vi "Install XNET and Scan If Needed.vi"(4 "XNET available":bool, 6 "xnet software to install":T1[](array[typedef]) {"component type" items=["standard", "hidden", "system", "unknown", "startup", "image"]}, 8 "error in (no error)":errorcluster, 9 "scan software to install":T1[](array[typedef]) {"component type" items=["standard", "hidden", "system", "unknown", "startup", "image"]}, 10 "software components on target":T1[](array[typedef]) {"component type" items=["standard", "hidden", "system", "unknown", "startup", "image"]}, 11 "Refnum in":refnum<k21>) -> (0 "error out":errorcluster, 3 "Refnum out":refnum<k21>)   [LabVIEW 2013]
uses:
  <vilib>/nisyscfg/Software 1.2.ctl
  <vilib>/nisyscfg/Component Type.ctl
  <vilib>/nisyscfg/Install or Uninstall Components.vi
  <vilib>/nisyscfg/Get Installed Components.vi
  <vilib>/nisyscfg/nisyscfg.lvlib
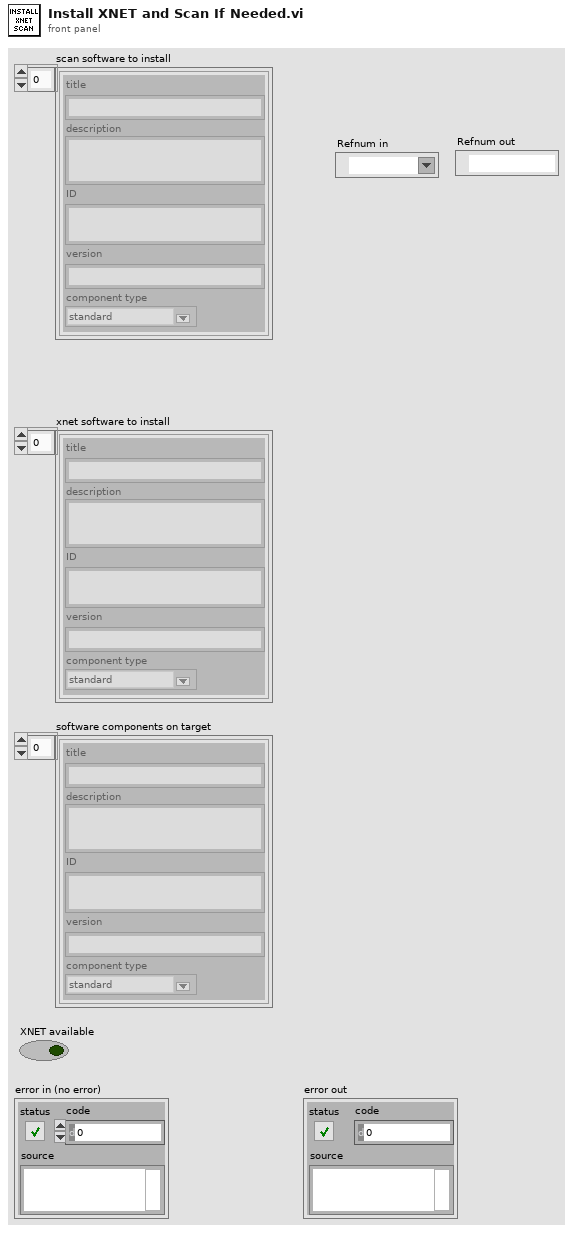
[diagram p1: front panel]
types:
  T1 = typedef "nisyscfg.lvlib/Software 1.2.ctl" = cluster{"title":string, "description":string, "ID":string, "version":string, "component type":T2}
  T2 = typedef "nisyscfg.lvlib/Component Type.ctl" = u32
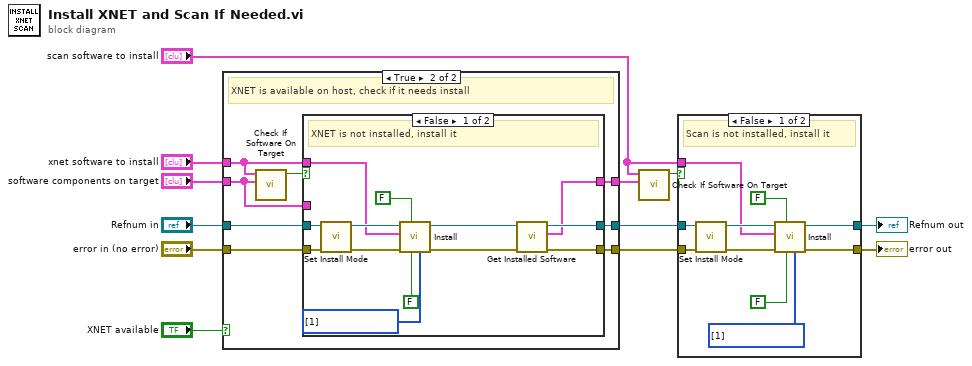
[diagram p0: block diagram]
diagram:
  n1 = case shown="True" "XNET available" {
    tunnel: "software components on target" -> [w13 w16]
    tunnel: "xnet software to install" -> [_ w20]
    tunnel: "error in (no error)" -> [w14 w22]
    tunnel: "Refnum in" -> [w15 w21]
    tunnel: [w14 w19] -> w9
    tunnel: [w15 w18] -> w6
    tunnel: [w13 w17] -> w1
    frame False {
      # "XNET not avilable on host, skip it"
    }
    frame True {
      # "XNET is available on host, check if it needs install"
      n2 = call "Check If Software On Target.vi"("installed software"=w16, "software to check"=w20) -> ("software installed"=w23:bool)  [unwired: 8 in, 1 out]
      n3 = case shown="False" w23 {
        tunnel: w22 -> [w36 w39]
        tunnel: w21 -> [w35 w38]
        tunnel: w20 -> [w31 _]
        tunnel: [w28 w39] -> w19
        tunnel: [w26 w38] -> w18
        tunnel: [w25 w37] -> w17
        tunnel: w16 -> [_ w37]
        frame False {
          w24 = u32[] [1] items=["Highest", "Exactly"] ("version selection (highest)")
          # "XNET is not installed, install it"
          n4 = call "Set Install Mode.vi"("error in"=w36, "session in"=w35) -> ("error out"=w33:errorcluster, "session out"=w34:refnum<k21>)  [unwired: 8 in]
          n5 = call-poly <vilib>:"Install.vi"("version selection (highest)"=w24, "auto-select dependencies (T)"=FALSE, "restart automatically (T)"=FALSE, "error in (no error)"=w33, "software components to install"=w31, "session in"=w34) -> ("error out"=w29:errorcluster, "session out"=w27:refnum<k21>)  [unwired: 3 in, 1 out]
          n6 = call-poly <vilib>:"Get Installed Software.vi"("error in (no error)"=w29, "session in"=w27) -> ("error out"=w28:errorcluster, "software components"=w25:T1[], "session out"=w26:refnum<k21>)  [unwired: 7 in]
        }
        frame True {
          # "XNET is installed"
        }
      }
    }
  }
  n7 = call "Check If Software On Target.vi"("installed software"=w1, "software to check"="scan software to install") -> ("software installed"=w7:bool)  [unwired: 8 in, 1 out]
  n8 = case shown="False" w7 {
    tunnel: w9 -> [w49 w51]
    tunnel: w6 -> [w48 w50]
    tunnel: "scan software to install" -> [w44 _]
    tunnel: [w42 w51] -> w11
    tunnel: [w41 w50] -> w12
    frame False {
      w40 = u32[] [1] items=["Highest", "Exactly"] ("version selection (highest)")
      # "Scan is not installed, install it"
      n9 = call "Set Install Mode.vi"("error in"=w49, "session in"=w48) -> ("error out"=w46:errorcluster, "session out"=w47:refnum<k21>)  [unwired: 8 in]
      n10 = call-poly <vilib>:"Install.vi"("version selection (highest)"=w40, "auto-select dependencies (T)"=FALSE, "restart automatically (T)"=FALSE, "error in (no error)"=w46, "software components to install"=w44, "session in"=w47) -> ("error out"=w42:errorcluster, "session out"=w41:refnum<k21>)  [unwired: 3 in, 1 out]
    }
    frame True {
      # "scan is installed"
    }
  }
  "Refnum out" <- w12
  "error out" <- w11
